vi "SSP - set value array STR.vi"(8 "error in (no error)":errorcluster, 11 "JSON string":string) -> (0 "error out":errorcluster, 3 "value":string)   [LabVIEW 2020, in "ui-testing.lvlib"]
doc: "copyright: Thomas Zilliox©"
uses:
  ui-testing.lvlib
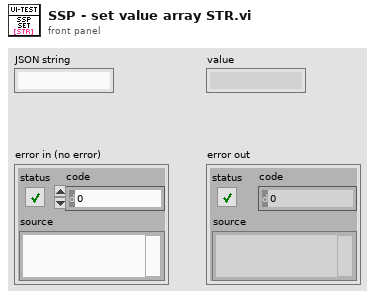
[diagram p1: front panel]
types:
  T1 = cluster{"control":string, "subpanel":string, "subsubpanel":string, "value":string[]}
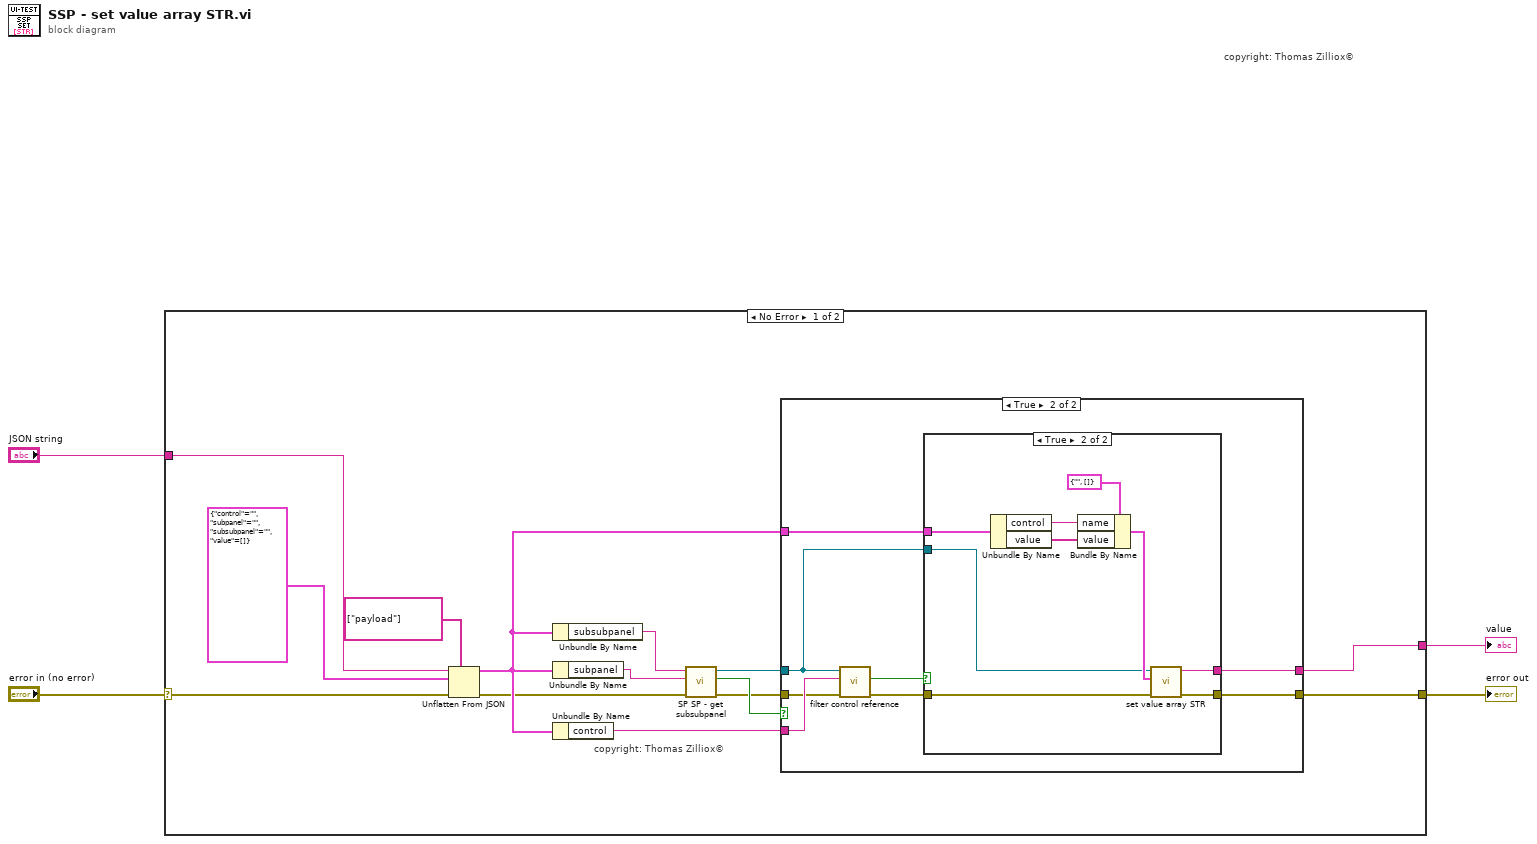
[diagram p0: block diagram]
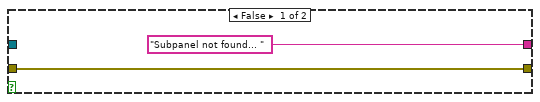
[diagram p2: hidden frame]
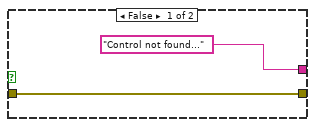
[diagram p3: hidden frame]
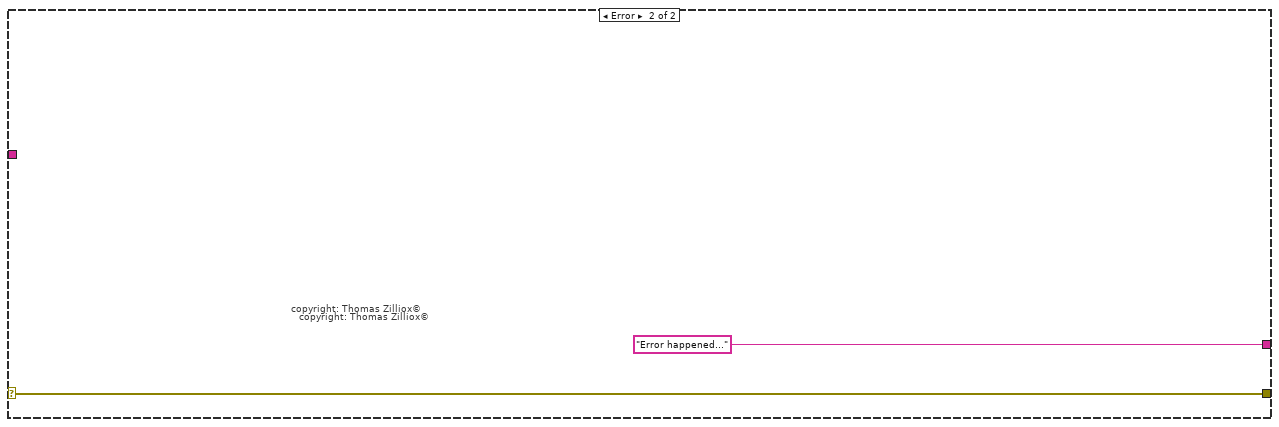
[diagram p4: hidden frame]
diagram:
  # "copyright: Thomas Zilliox©"
  n1 = case shown="No Error" "error in (no error)" {
    selector: "error in (no error)" -> [w15 w41]
    tunnel: "JSON string" -> [w17 _]
    tunnel: [w16 w41] -> w3
    tunnel: [w14 "Error happened..."] -> w1
    frame No Error {
      # "copyright: Thomas Zilliox©"
      n2 = Unflatten From JSON(path=string[] ["payload"], JSON string=w17, type and defaults=T1 {"control"="", "subpanel"="", "subsubpanel"="", "value"=[]}, error in (no error)=w15) -> (value=w11:T1, error out=w6:errorcluster)  [unwired: 3 in]
      n3 = Unbundle By Name(w11) -> ("subsubpanel"=w9:string)
      n4 = Unbundle By Name(w11) -> ("subpanel"=w10:string)
      n5 = Unbundle By Name(w11) -> ("control"=w12:string)
      n6 = call "SP SP - get subsubpanel.vi"("error in (no error)"=w6, "subpanel"=w10, "subsubpanel"=w9) -> ("error out"=w5:errorcluster, "SubSubPanel found"=w8:bool, "SubSubPanel VI"=w7:refnum<vi>)  [unwired: 5 in, 1 out]
      n7 = case shown="True" w8 {
        tunnel: [w20 w28] -> w16
        tunnel: w7 -> [_ w25]
        tunnel: w5 -> [w20 w23]
        tunnel: w12 -> [_ w24]
        tunnel: ["Subpanel not found... " ("result string") w27] -> w14
        tunnel: w11 -> [_ w26]
        frame False {
        }
        frame True {
          n8 = call "filter control reference.vi"("error in (no error)"=w23, "Control label"=w24, "VI (Caller)"=w25) -> ("error out"=w21:errorcluster, "Control found"=w22:bool)  [unwired: 6 in, 1 out]
          n9 = case shown="True" w22 {
            tunnel: w21 -> [w30 w33]
            tunnel: [w30 w31] -> w28
            tunnel: ["Control not found..." ("result string") w32] -> w27
            tunnel: w26 -> [_ w35]
            tunnel: w25 -> [_ w34]
            frame False {
            }
            frame True {
              n10 = Unbundle By Name(w35) -> ("control"=w36:string, "value"=w37:string[])
              n11 = Bundle By Name(cluster=cluster{"name":string, "value":string[]} {"name"="", "value"=[]} ("Payload"), "name"=w36, "value"=w37) -> (w38:cluster{"name":string, "value":string[]})
              n12 = call "set value array STR.vi"("error in (no error)"=w33, "Payload"=w38, "VI Ref"=w34) -> ("error out"=w31:errorcluster, "return value"=w32:string)  [unwired: 7 in]
            }
          }
        }
      }
    }
    frame Error {
      # "copyright: Thomas Zilliox©"
      # "copyright: Thomas Zilliox©"
    }
  }
  "error out" <- w3
  "value" <- w1
